vi "p10 decodificador imagenes.vi"() -> ()   [LabVIEW 2013]
panel:
  out "Numeric":i32
  in  "path to BMP file 3":path
  in  "path to BMP file":path
  in  "Array":bool[](array[boolean])
  out "new picture 2":picture
  out "new picture":picture
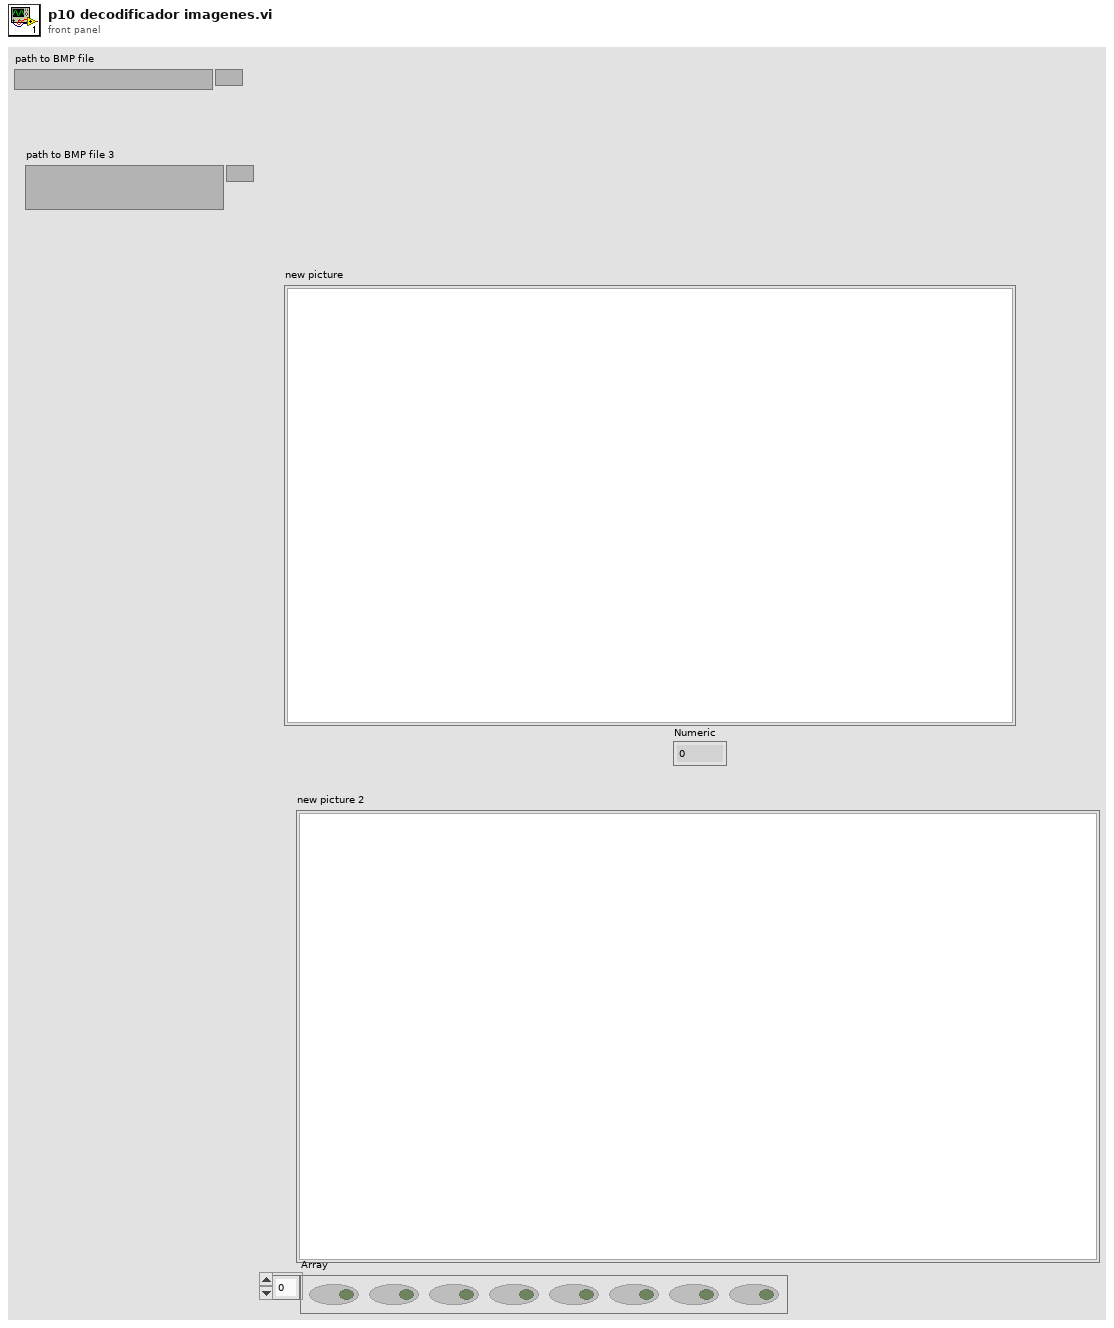
[diagram p1: front panel]
types:
  T1 = typedef "imagedata.ctl" = cluster{"image type":i32, "image depth":i32, "image":u8[], "mask":u8[], "colors":u32[], "Rectangle":cluster{"left":i16, "top":i16, "right":i16, "bottom":i16}}
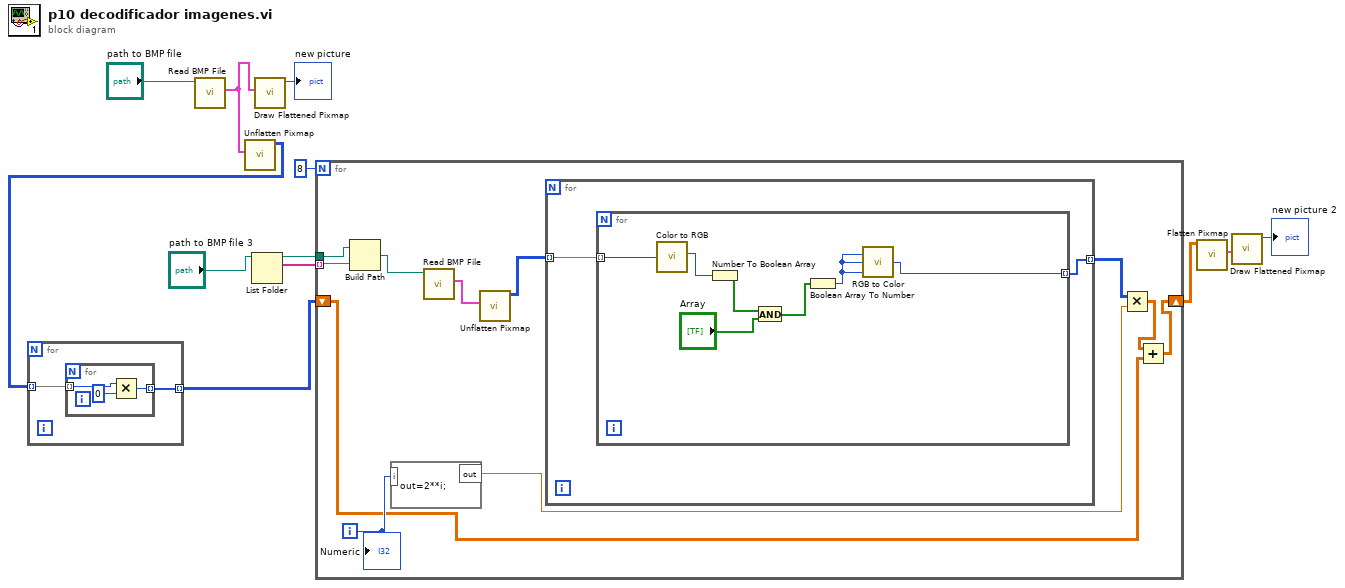
[diagram p0: block diagram]
diagram:
  n1 = call <vilib>:"Read BMP File.vi"("path to BMP file"="path to BMP file") -> ("image data"=w7:T1)  [unwired: 8 in, 2 out]
  n2 = call <vilib>:"Unflatten Pixmap.vi"("image data"=w7) -> ("24-bit pixmap"=w2:u32[][])  [unwired: 4 in, 6 out]
  n3 = for {
    tunnel: w2 -> [w14] mode=indexing
    tunnel: [w13] -> w1 mode=indexing
    n4 = for {
      tunnel: w14 -> [w17] mode=indexing
      tunnel: [w15] -> w13 mode=indexing
      n5 = Multiply(x=w17, y=u32 0) -> (x*y=w15:u32)
    }
  }
  n6 = List Folder(path="path to BMP file 3") -> (path out=w5:path, filenames=w4:string[])  [unwired: 3 in, 2 out]
  n7 = call <vilib>:"Draw Flattened Pixmap.vi"("image data"=w7) -> ("new picture"=→"new picture":picture)  [unwired: 8 in]
  n8 = for {
    N: 8 -> [_]
    tunnel: w5 -> [w24]
    tunnel: w4 -> [w23] mode=indexing
    shift-right: [w18] -> w3
    shift-left: w1 -> [w20]
    i -> [w26]
    n9 = Build Path(base path=w24, name or relative path=w23) -> (appended path=w22:path)
    n10 = formula code="out=2**i;"("i"=w26) -> ("out"=w25:dbl)
    n11 = call <vilib>:"Read BMP File.vi"("path to BMP file"=w22) -> ("image data"=w28:T1)  [unwired: 8 in, 2 out]
    n12 = call <vilib>:"Unflatten Pixmap.vi"("image data"=w28) -> ("24-bit pixmap"=w27:u32[][])  [unwired: 4 in, 6 out]
    n13 = for {
      tunnel: w27 -> [w30] mode=indexing
      tunnel: [w29] -> w21 mode=indexing
      n14 = for {
        tunnel: w30 -> [w33] mode=indexing
        tunnel: [w32] -> w29 mode=indexing
        n15 = call <vilib>:"Color to RGB.vi"("Color"=w33) -> ("R"=w37:u8)  [unwired: 3 out]
        n16 = Number To Boolean Array(number=w37) -> (Boolean array=w36:bool[])
        n17 = And(x=w36, y="Array") -> (x .and. y?=w34:bool[])
        n18 = Boolean Array To Number(Boolean array=w34) -> (number=w31:u32)
        n19 = call <vilib>:"RGB to Color.vi"("B"=w31, "G"=w31, "R"=w31) -> ("Color"=w32:u32)
      }
    }
    n20 = Multiply(x=w21, y=w25) -> (x*y=w19:dbl[][])
    n21 = Add ("Add.vi")(x=w19, y=w20) -> (x+y=w18:dbl[][])
    "Numeric" <- w26
  }
  n22 = call <vilib>:"Flatten Pixmap.vi"("24-bit pixmap"=w3) -> ("image data"=w11:T1)  [unwired: 10 in]
  n23 = call <vilib>:"Draw Flattened Pixmap.vi"("image data"=w11) -> ("new picture"=→"new picture 2":picture)  [unwired: 8 in]
